vi "HoloPy_set_parameters.vi"(8 "error in (no error)":errorcluster, 10 "ParametersIN":T1={"Holo parameters"={"wavelength"=0.0, "optical index"=0.0, "Holo size X"=0, "Holo size Y"=0, "pixel size"=0.0, "objective magnification"=0.0}, "propagation"={"distance ini"=0.0, "number of planes"=0, "step"=0.0}, "Fourier BP filter (pix)"={"High pass (0=none)"=0.0, "Low Pass (0=none)"=0.0}, "Focus"={"Type"=enum."CUSTOM", "Sum size"=15}, "CCL parameters"={"Threshold ( N x Standard deviation)"=0.0, "Connectivity"=enum."6", "min voxel"=0.0, "max voxel"=0.0}} {"Holo parameters"."Holo size X" format="%.0g"; "Holo parameters"."pixel size" format="%#_6e"; "Holo parameters"."wavelength" format="%#_6e"; "CCL parameters"."max voxel" min=0.0 max=0.0; "CCL parameters"."min voxel" min=1.0 max=100.0; "CCL parameters"."Threshold ( N x Standard deviation)" min=1.0 max=100.0}, 11 "session in":refnum<k35>) -> (0 "error out":errorcluster, 2 "return value":string, 3 "Refnum out":refnum<k35>)   [LabVIEW 2025, in "holoTracker.lvlib"]
uses:
  holoTracker.lvlib
  subVis/all_treatment_parameters.ctl
  subVis/HologramInfo.ctl
  CCL_parameters.ctl
panel:
  # "wavelenght, optical_index, image_size_X, image_size_Y, pixel_size, magnification = holo_info\n\n    propag_param, focus_param, binarisation_param, CCL_param = analyse_parameters\n    distance_ini, nb_plane, propag_step, filter = propag_param\n    high_pass_filter, low_pass_filter = filter\n    #focus parameters unpacking\n    focus_type, sum_size = focus_param\n    #binarisation parameters unpacking\n    nbStdVarThreshold, threshold_target = binarisation_param\n    #CCL parameters unpacking\n    n_connectivity, min_voxel, max_voxel = CCL_param"
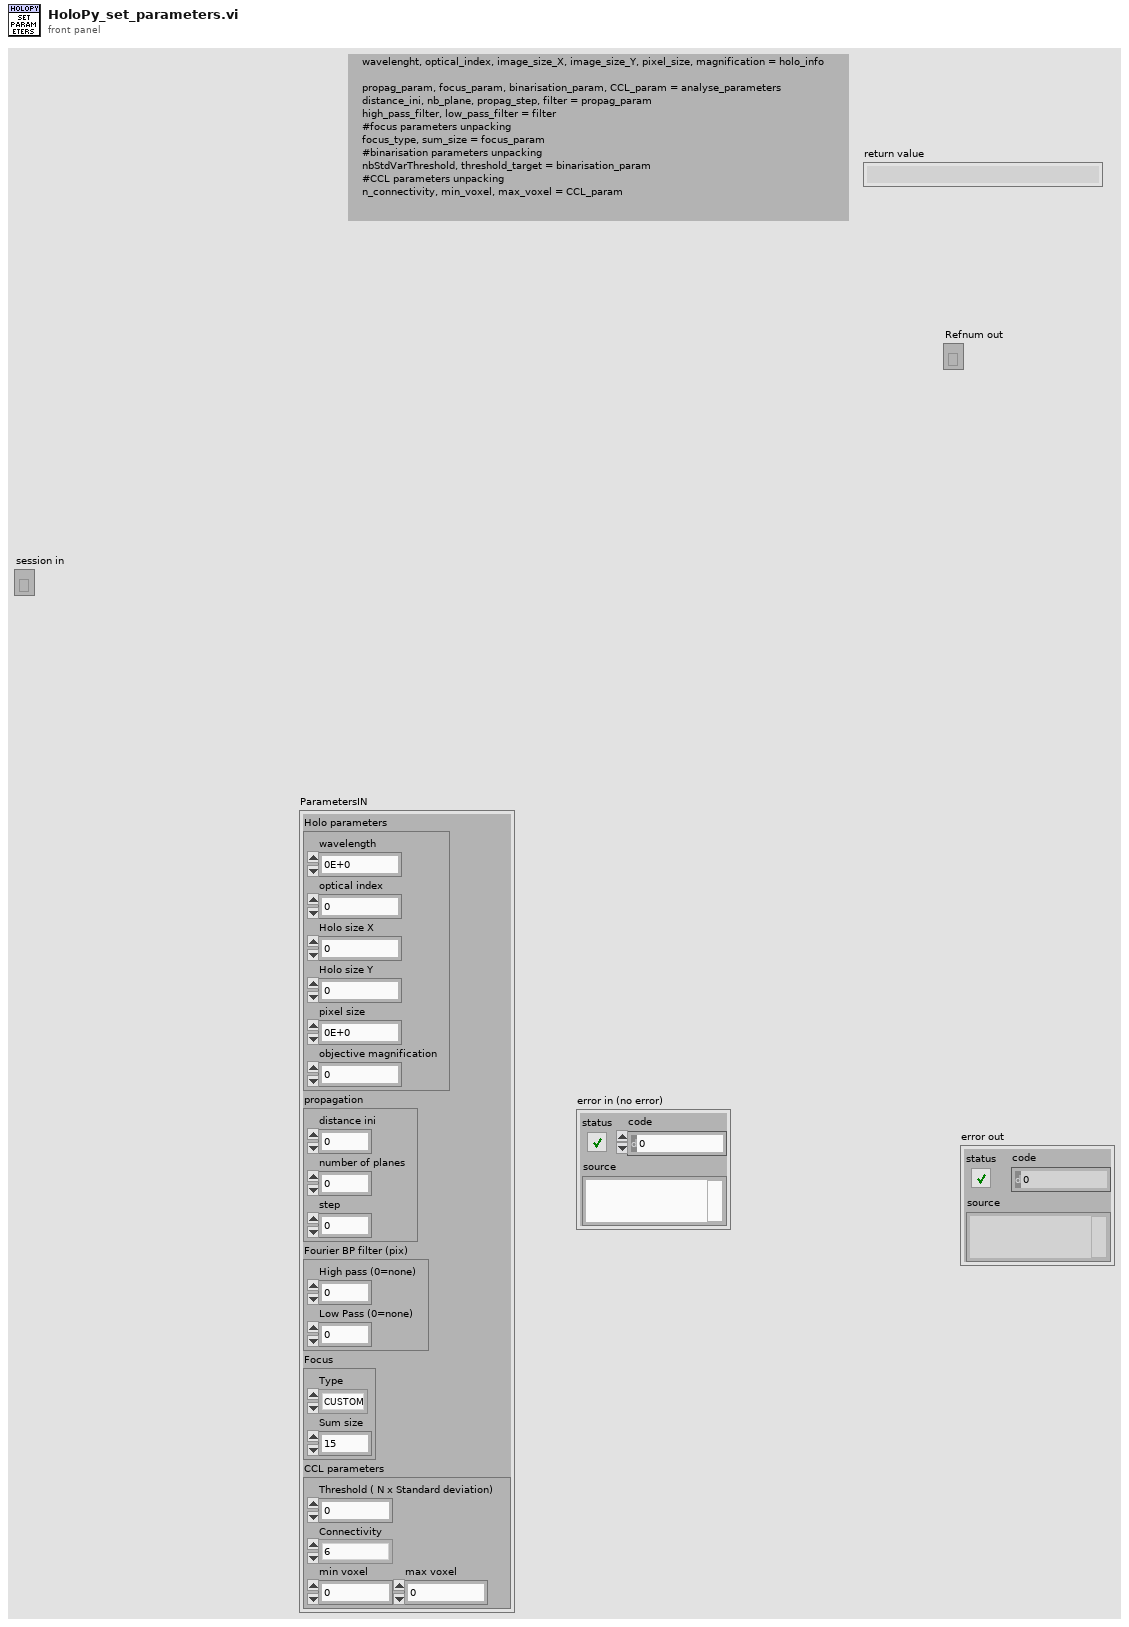
[diagram p1: front panel]
types:
  T1 = typedef "all_treatment_parameters.ctl" = cluster{"Holo parameters":T2, "propagation":cluster{"distance ini":dbl, "number of planes":i32, "step":dbl}, "Fourier BP filter (pix)":cluster{"High pass (0=none)":dbl, "Low Pass (0=none)":dbl}, "Focus":cluster{"Type":enum16{"SUM_OF_INTENSITY", "SUM_OF_LAPLACIAN", "SUM_OF_VARIANCE", "TENENGRAD", "CUSTOM"}, "Sum size":i32}, "CCL parameters":T3}
  T2 = typedef "holoTracker.lvlib/HologramInfo.ctl" = cluster{"wavelength":sgl, "optical index":sgl, "Holo size X":i32, "Holo size Y":i32, "pixel size":sgl, "objective magnification":sgl}
  T3 = typedef "CCL_parameters.ctl" = cluster{"Threshold ( N x Standard deviation)":dbl, "Connectivity":enum16{"6", "18", "26"}, "min voxel":dbl, "max voxel":dbl}
  T4 = cluster{"distance ini":dbl, "number of planes":i32, "step":dbl}
  T5 = cluster{"High pass (0=none)":dbl, "Low Pass (0=none)":dbl}
  T6 = cluster{"Type":enum16{"SUM_OF_INTENSITY", "SUM_OF_LAPLACIAN", "SUM_OF_VARIANCE", "TENENGRAD", "CUSTOM"}, "Sum size":i32}
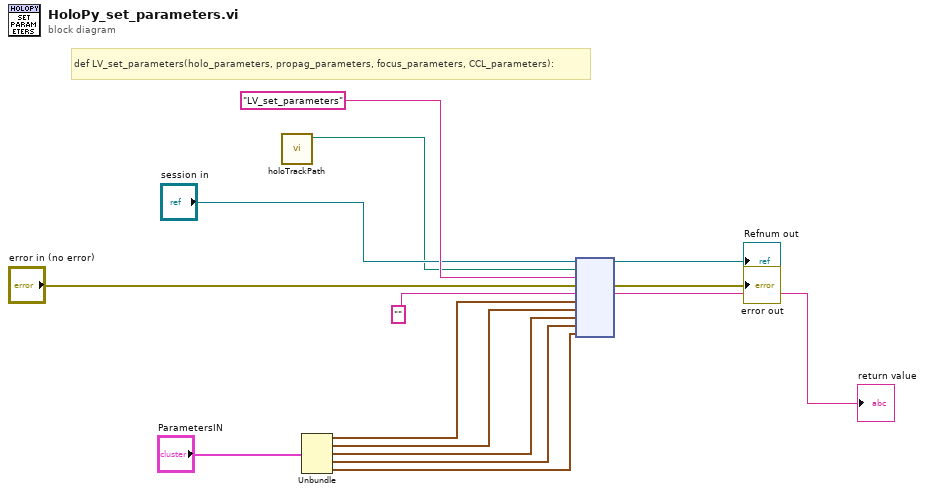
[diagram p0: block diagram]
diagram:
  # "def LV_set_parameters(holo_parameters, propag_parameters, focus_parameters, CCL_parameters):"
  n1 = call "holoTrackPath.vi"() -> ("appended path"=w8:path)  [unwired: 11 in]
  n2 = Unbundle("ParametersIN") -> ("Holo parameters"=w6:T2, "propagation"=w5:T4, "Fourier BP filter (pix)"=w4:T5, "Focus"=w3:T6, "CCL parameters"=w2:T3)
  n3 = node("session in", w8, "LV_set_parameters" ("function name"), "error in (no error)", "", w6, w5, w4, w3, w2) -> (→"Refnum out":refnum<k35>, →"error out":errorcluster, →"return value":string)  [unwired: 5 in, 2 out]
